vi "MD5 (String).vi"(10 "message":string) -> (2 "MD5 hash":string)   [LabVIEW 2013, in "MD5.lvlib"]
uses:
  MD5.lvlib
  MD5.lvclass
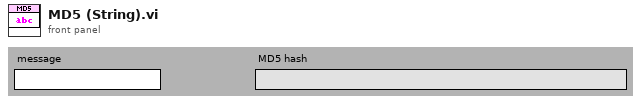
[diagram p1: front panel]
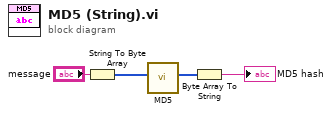
[diagram p0: block diagram]
diagram:
  n1 = String To Byte Array(string="message") -> (unsigned byte array=w2:u8[])
  n2 = call "MD5.vi"("data"=w2) -> ("MD5 hash"=w3:u8[])  [unwired: 10 in]
  n3 = Byte Array To String(unsigned byte array=w3) -> (string=→"MD5 hash":string)
